vi "AalborgDFCErrorCodes.vi"(4 "Error Code":string) -> (1 "Error Description":string)   [LabVIEW 2015]
panel:
  in  "Aalborg DFC Error Strings":string="Programming Reference \nError Code Fault \n0 No Error \nData Errors \nError#1 Invalid Command. \nError#2 Invalid number of arguments. \nError#3 Hardware for requested function is not installed (not available). \nError#4 Wrong number of characters in the argument. \nError#5 Attempt to Alter Write Protected Area in the EEPROM. \nError#6 Proper Command or Argument is not found. \nError#7 Wrong value of the Argument. \nError#8 Wrong Command. \nError#9 Reserved. \nError#10 Argument out of range. \nError#11 Auto ZERO in Progress. "
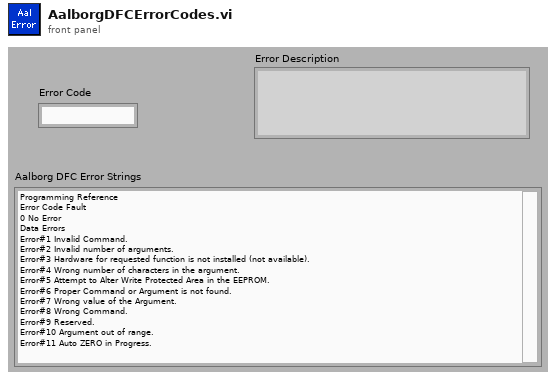
[diagram p1: front panel]
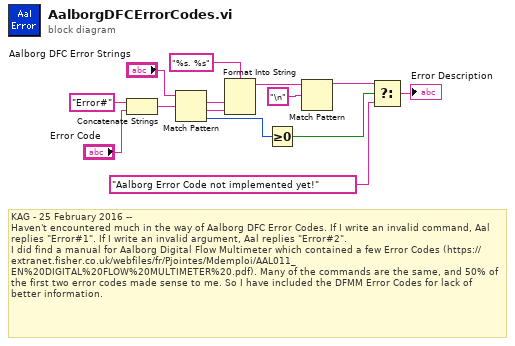
[diagram p0: block diagram]
diagram:
  # "KAG - 25 February 2016 --\nHaven't encountered much in the way of Aalborg DFC Error Codes. If I write an invalid command, Aal replies \"Error#1\". If I write an invalid argument, Aal replies \"Error#2\".\nI did find a manual for Aalborg Digital Flow Multimeter which contained a few Error Codes (https://extranet.fisher.co.uk/webfiles/fr/Pjointes/Mdemploi/AAL011_EN%20DIGITAL%20FLOW%20MULTIMETER%20.pdf). Many of the commands are the same, and 50% of the first two error codes made sense to me. So I have included the DFMM Error Codes for lack of better information."
  n1 = Concatenate Strings("Error#", "Error Code") -> (w5:string)
  n2 = Match Pattern(string="Aalborg DFC Error Strings", regular expression=w5) -> (match substring=w4:string, after substring=w3:string, offset past match=w12:i32)  [unwired: 2 out]
  n3 = Format Into String(format string="%s. %s", w4, w3) -> (resulting string=w1:string)  [unwired: 2 in, 1 out]
  n4 = Greater Or Equal To 0?(x=w12) -> (x >= 0?=w11:bool)
  n5 = Match Pattern(string=w1, regular expression="\n") -> (before substring=w10:string)  [unwired: 4 out]
  n6 = Select(t=w10, s=w11, f="Aalborg Error Code not implemented yet!") -> (s? t:f=→"Error Description":string)
